vi "error_messages.vi"(8 "error in (no error)":errorcluster) -> ()   [LabVIEW 2015]
uses:
  <vilib>/Utility/error.llb/DialogType.ctl
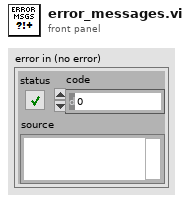
[diagram p1: front panel]
types:
  T1 = typedef "DialogType.ctl" = u16
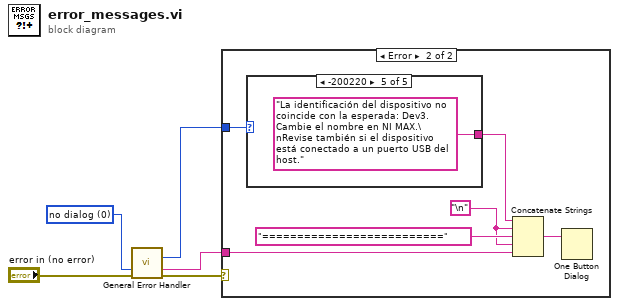
[diagram p0: block diagram]
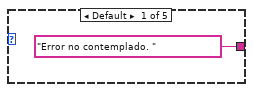
[diagram p3: hidden frame]
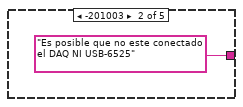
[diagram p4: hidden frame]
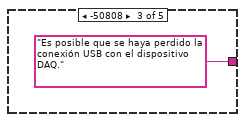
[diagram p5: hidden frame]
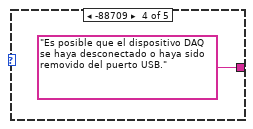
[diagram p6: hidden frame]
diagram:
  w2 = T1 0 items=["no dialog", "OK message", "continue or stop message", "OK message + warnings", "continue/stop + warnings"] ("type of dialog (OK msg:1)")
  n1 = call <vilib>:"General Error Handler.vi"("type of dialog (OK msg:1)"=w2, "error in (no error)"="error in (no error)") -> ("code out"=w4:i32, "message"=w5:string, "error out"=w3:errorcluster)  [unwired: 9 in, 2 out]
  n2 = case shown="Error" w3 {
    tunnel: w4 -> [_ w11]
    tunnel: w5 -> [_ w9]
    frame No Error {
    }
    frame Error {
      w6 = "\n"
      n3 = case shown="-200220" w11 {
        tunnel: ["Error no contemplado. " "Es posible que no este conectado el DAQ NI USB-6525" "Es posible que se haya perdido la conexión USB con el dispositivo DAQ." "Es posible que el dispositivo DAQ se haya desconectado o haya sido removido del puerto USB." "La identificación del dispositivo no coincide con la esperada: Dev3. Cambie el nombre en NI MAX.\nRevise también si el dispositivo está conectado a un puerto USB del host."] -> w10
        frame Default {
        }
        frame -201003 {
        }
        frame -50808 {
        }
        frame -88709 {
        }
        frame -200220 {
        }
      }
      n4 = Concatenate Strings(w10, w6, "==========================", w6, w9) -> (w8:string)
      n5 = One Button Dialog(message=w8) -> ()  [unwired: 1 in, 1 out]
    }
  }
